vi "testCode.vi"() -> ()   [LabVIEW 2022 SP3]
uses:
  Switch_MotorP5.lvclass
  C:/Projects/Medulla/ViPER/Examples/Flux_Capacitor_Tester/Components/ViPER.lvlibp/ViPER.lvclass
  Components/ViPER.lvlibp/ViPER.lvclass
panel:
  in  "Connect":bool
  in  "channel 1":string caption="Route"
  in  "route":bool
  out "Value":dbl
  in  "stop":bool
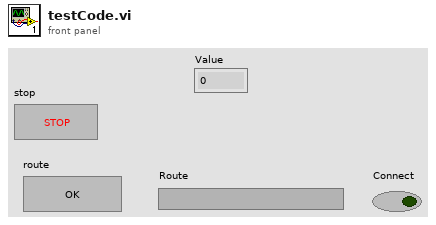
[diagram p1: front panel]
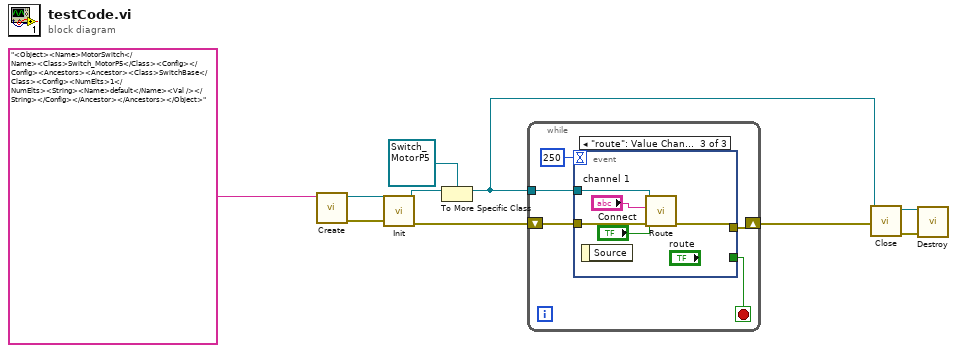
[diagram p0: block diagram]
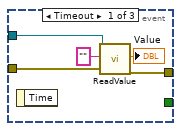
[diagram p2: hidden frame]
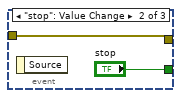
[diagram p3: hidden frame]
diagram:
  n1 = call "Create.vi"("Config XML"="<Object><Name>MotorSwitch</Name><Class>Switch_MotorP5</Class><Config></Config><Ancestors><Ancestor><Class>SwitchBase</Class><Config><NumElts>1</NumElts><String><Name>default</Name><Val /></String></Config></Ancestor></Ancestors></Object>") -> ("error out"=w9:errorcluster, "reference out"=w10:refnum<class "ViPER.lvclass">)  [unwired: 9 in]
  n2 = call-dynamic "Init.vi"("error in (no error)"=w9, "reference in"=w10) -> ("error out"=w6:errorcluster, "reference out"=w8:refnum<class "ViPER.lvclass">)  [unwired: 8 in]
  n3 = To More Specific Class(target class=refnum<class "Switch_MotorP5.lvclass"> refnum ("reference in"), reference=w8) -> (specific class reference=w5:refnum<class "Switch_MotorP5.lvclass">)  [unwired: 1 in, 1 out]
  n4 = while {
    tunnel: w5 -> [w14]
    shift-right: [w12] -> w4
    shift-left: w6 -> [w13]
    stop <- w11 stop-if-true
    n5 = event shown="[2] \"route\": Value Change" {
      selector: _ -> [_ _ _]
      dyn-events: _ -> [_ _ _]
      timeout: 250 -> [_ _ _]
      tunnel: w14 -> [w20 _ w25]
      tunnel: w13 -> [w19 w22 w27]
      tunnel: [w17 w22 w26] -> w12
      tunnel: [_ "stop" _] -> w11
      event Timeout {
        n6 = event-data() -> ()  [unwired: 1 in, 1 out]
        n7 = call-dynamic "ReadValue.vi"("reference in"=w20, "Name"="", "error in (no error)"=w19) -> ("Value"=→"Value":dbl, "error out"=w17:errorcluster)  [unwired: 14 in, 1 out]
      }
      event "stop": Value Change {
        n8 = event-data() -> ()  [unwired: 1 in, 1 out]
      }
      event "route": Value Change {
        n9 = event-data() -> ()  [unwired: 1 in, 1 out]
        n10 = call-dynamic "Route.vi"("error in (no error)"=w27, "Connect"="Connect", "channel 1"="channel 1", "reference in"=w25) -> ("error out"=w26:errorcluster)  [unwired: 6 in, 1 out]
      }
    }
  }
  n11 = call-dynamic "Close.vi"("error in (no error)"=w4, "reference in"=w5) -> ("error out"=w2:errorcluster, "reference in"=w3:refnum<class "Switch_MotorP5.lvclass">)  [unwired: 8 in]
  n12 = call "Destroy.vi"("error in (no error)"=w2, "reference in"=w3) -> ()  [unwired: 9 in, 1 out]
